vi "easing_QuadOut.vi"(9 "distance":dbl, 10 "interval (10 ms)":dbl, 11 "time":dbl) -> (3 "current pos":dbl)   [LabVIEW 2023]
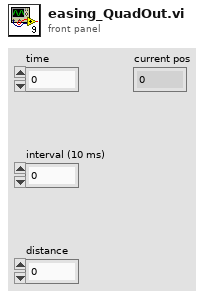
[diagram p1: front panel]
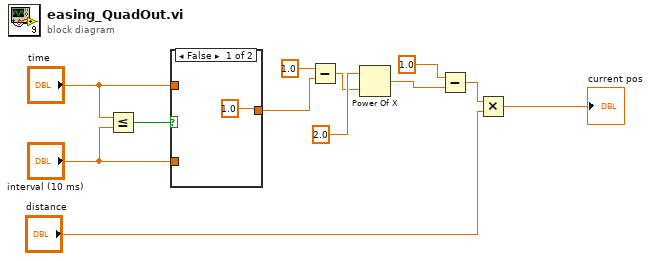
[diagram p0: block diagram]
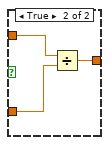
[diagram p2: hidden frame]
diagram:
  n1 = Less Or Equal?(x="time", y="interval (10 ms)") -> (x <= y?=w1:bool)
  n2 = case shown="False" w1 {
    tunnel: [1.0 ("y") w16] -> w8
    tunnel: "interval (10 ms)" -> [_ w15]
    tunnel: "time" -> [_ w14]
    frame False {
    }
    frame True {
      n3 = Divide(x=w14, y=w15) -> (x/y=w16:dbl)
    }
  }
  n4 = Subtract(x=1.0 ("y"), y=w8) -> (x-y=w4:dbl)
  n5 = Power Of X(1:w4, 2:2.0 ("y")) -> (0:w9:dbl)
  n6 = Subtract(x=1.0 ("y"), y=w9) -> (x-y=w10:dbl)
  n7 = Multiply(x=w10, y="distance") -> (x*y=→"current pos":dbl)
